vi "Is Open.vi"(8 "error in (no error)":errorcluster, 11 "TCP Client in":refnum<class "TCP Client.lvclass">) -> (0 "error out":errorcluster, 2 "Is Open":bool, 3 "TCP Client out":refnum<class "TCP Client.lvclass">)   [LabVIEW 2020, in "Stream-TCP.lvlib" / "TCP Client.lvclass"]
uses:
  TCP Client.lvclass
  C:/Program Files (x86)/National Instruments/LabVIEW 2020/vi.lib/IlluminatedG/lv-stream/Connection/Connection.lvclass
  <vilib>/IlluminatedG/lv-stream/Connection/State.ctl
  <vilib>/IlluminatedG/lv-stream/Connection/Connection.lvclass
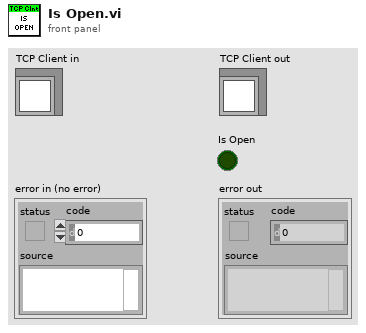
[diagram p1: front panel]
types:
  T1 = typedef "Stream.lvlib/Connection.lvclass/State.ctl" = enum16{"Closed", "Idle", "Connecting", "Connected", "Shutdown"}
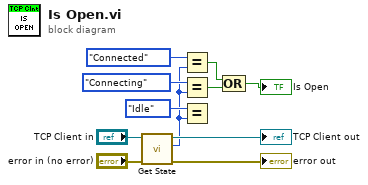
[diagram p0: block diagram]
diagram:
  n1 = call <vilib>:"Get State.vi"("error in (no error)"="error in (no error)", "Connection in"="TCP Client in") -> ("error out"=→"error out":errorcluster, "State"=w2:T1, "Connection out"=→"TCP Client out":refnum<class "TCP Client.lvclass">)  [unwired: 7 in]
  n2 = Equal?(x=State."Connected", y=w2) -> (x = y?=w1:bool)
  n3 = Equal?(x=State."Connecting", y=w2) -> (x = y?=w5:bool)
  n4 = Equal?(x=State."Idle", y=w2) -> ()  [unwired: 1 out]
  n5 = Compound Arithmetic op=OR(w1, w5) -> (→"Is Open":bool)
